vi "Write waveform 1D.vi"(4 "Channel":string="wave", 6 "Arr notes":string[](array[string]), 8 "error in (no error)":errorcluster, 10 "Arr waveform":waveform(dbl)[](array[waveform])) -> (0 "error out":errorcluster)   [LabVIEW 2019]
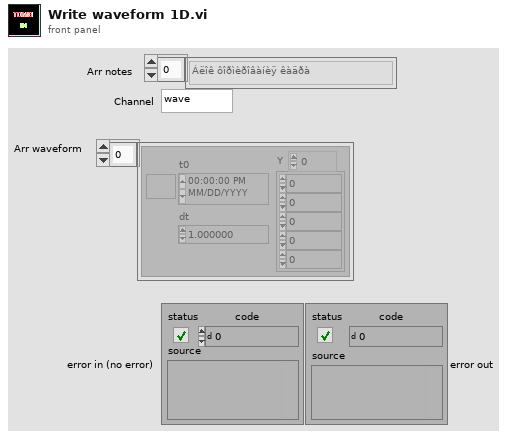
[diagram p1: front panel]
types:
  T1 = enum16{"open", "open or create", "create or replace", "create", "open (read-only)"}
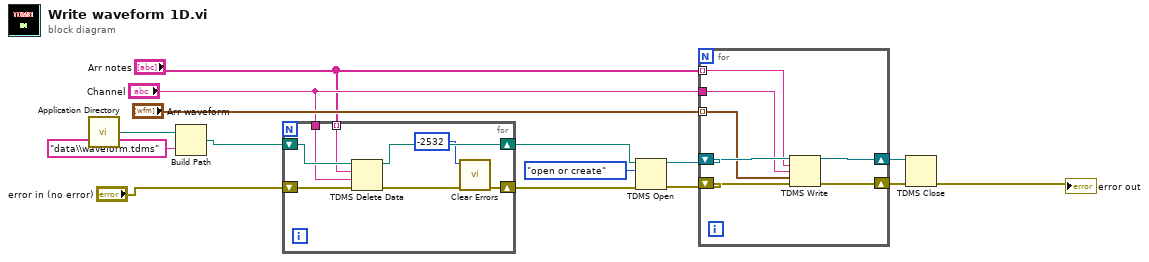
[diagram p0: block diagram]
diagram:
  n1 = call <vilib>:"Application Directory.vi"() -> ("Application Directory"=w14:path)
  n2 = Build Path(base path=w14, name or relative path="data\\waveform.tdms") -> (appended path=w4:path)
  n3 = for {
    shift-right: [w16] -> w5
    shift-left: "error in (no error)" -> [w23]
    shift-right: [w21] -> w3
    shift-left: w4 -> [w22]
    tunnel: "Channel" -> [w20]
    tunnel: "Arr notes" -> [w19] mode=indexing
    n4 = TDMS Delete Data(8:w23, 9:w20, 10:w19, 11:w22) -> (0:w17:errorcluster, 3:w21:path)  [unwired: 3 in]
    n5 = call <vilib>:"Clear Errors.vi"("error in (no error)"=w17, "specific error code to clear (0: all)"=-2532) -> ("error out"=w16:errorcluster)  [unwired: 4 in, 1 out]
  }
  n6 = TDMS Open(8:w5, 10:T1."open or create" ("operation (0:open)"), 11:w3) -> (0:w11:errorcluster, 3:w12:refnum<k34>)  [unwired: 4 in]
  n7 = for {
    tunnel: "Arr notes" -> [w28] mode=indexing
    tunnel: "Arr waveform" -> [w27] mode=indexing
    tunnel: "Channel" -> [w26]
    shift-right: [w25] -> w9
    shift-left: w12 -> [w30]
    shift-right: [w24] -> w8
    shift-left: w11 -> [w29]
    n8 = TDMS Write(0:w30, 5:w28, 7:w26, 9:w27, 11:w29) -> (4:w25:refnum<k34>, 15:w24:errorcluster)  [unwired: 1 in, 2 out]
  }
  n9 = TDMS Close(8:w8, 11:w9) -> (0:→"error out":errorcluster)  [unwired: 1 out]
